vi "9602 Mandatory field missing for ObjectType--error.vi"(8 "error in":errorcluster, 10 "Field Name":string, 11 "Object Type Base":refnum<class "Object Type Base.lvclass">) -> (0 "error out":errorcluster)   [LabVIEW 2024, in "Electronic Datasheet.lvlib"]
uses:
  Electronic Datasheet.lvlib
  Object Type/Object Type Base.lvclass
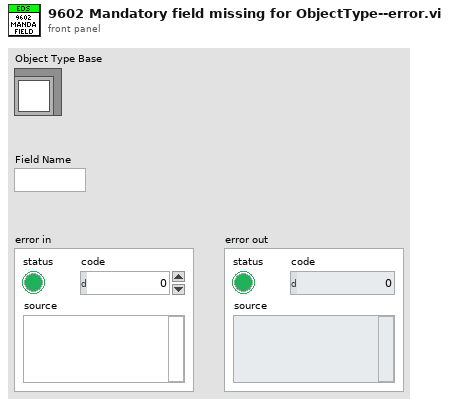
[diagram p1: front panel]
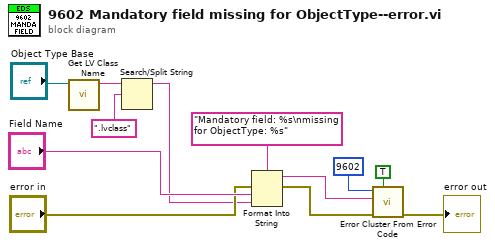
[diagram p0: block diagram]
diagram:
  n1 = call <vilib>:"Get LV Class Name.vi"("object"="Object Type Base") -> ("class name"=w3:string)  [unwired: 9 in, 1 out]
  n2 = Search/Split String(string=w3, search string/char (-)=".lvclass") -> (substring before match=w1:string)  [unwired: 1 in, 2 out]
  n3 = Format Into String(format string="Mandatory field: %s\nmissing for ObjectType: %s", error in="error in", "Field Name", w1) -> (resulting string=w8:string, error out=w5:errorcluster)  [unwired: 1 in]
  n4 = call <vilib>:"Error Cluster From Error Code.vi"("show call chain? (False)"=TRUE, "error in (no error)"=w5, "error message (\"\")"=w8, "error code (0)"=9602) -> ("error out"=→"error out":errorcluster)  [unwired: 5 in]
